vi "Variable@SDiff__Parameter.vi"(1 "ParamterIn":string) -> (0 "ParamterOut":string)   [LabVIEW 2020]
panel:
  out "f":i32
  in  "Var2":string(combo)
  in  "Section":string(combo)
  in  "Var1":string(combo)
  in  "ParameterName":string(combo)
  in  "Confirm":bool
  # "Variable@SUnion $Variable,$Var1,$Var2(,$Section)"
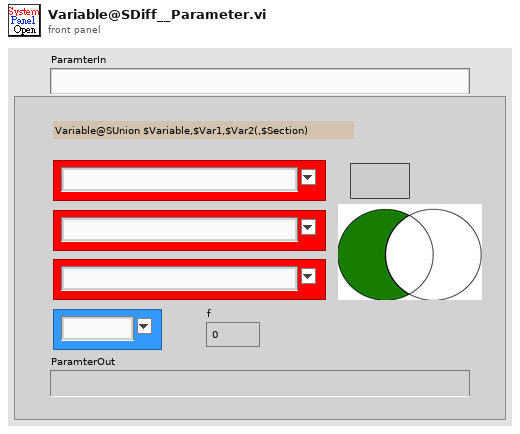
[diagram p1: front panel]
types:
  T1 = enum16{"Get", "Init", "Set", "Delete", "GetElement", "Inc", "Dec", "ReName"}
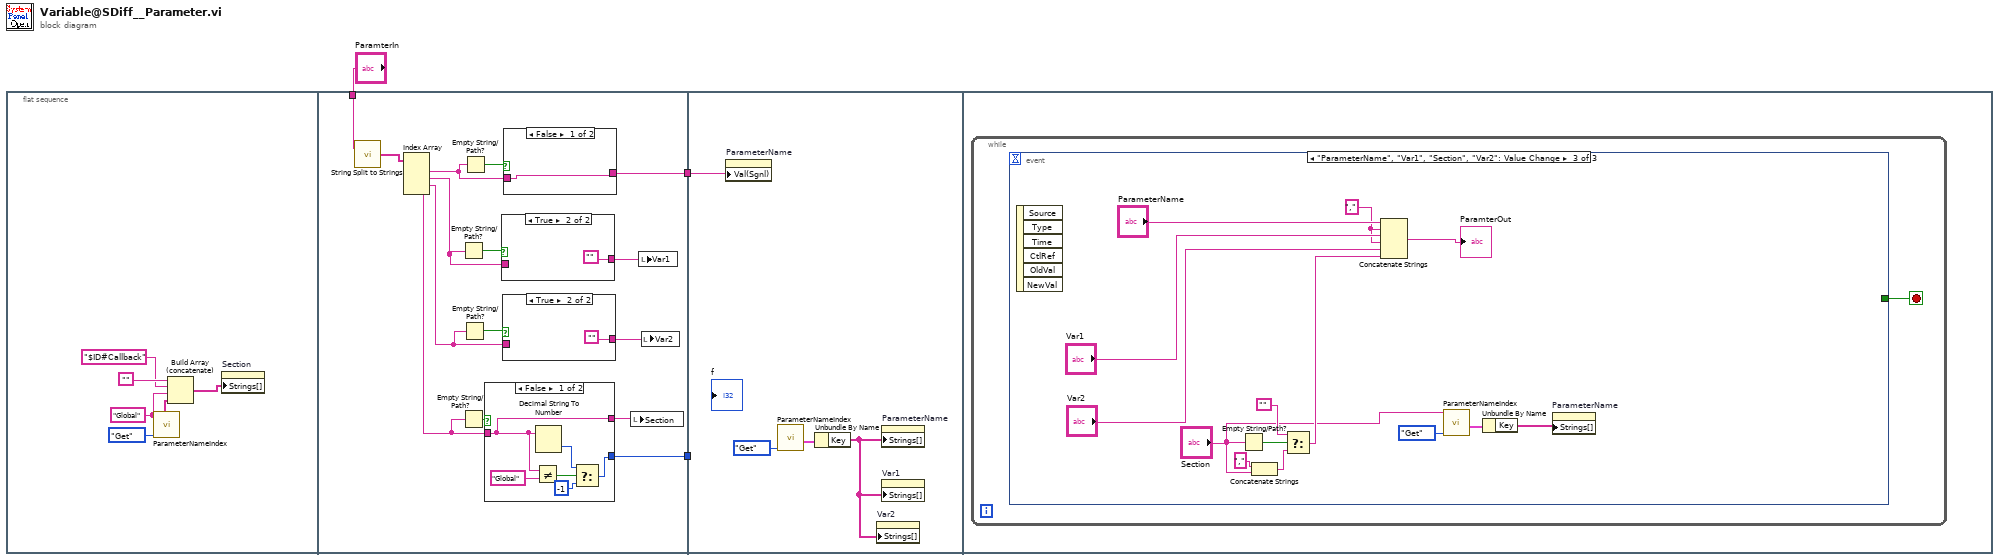
[diagram p0: block diagram]
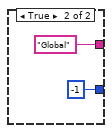
[diagram p3: hidden frame]
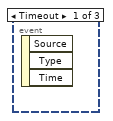
[diagram p6: hidden frame]
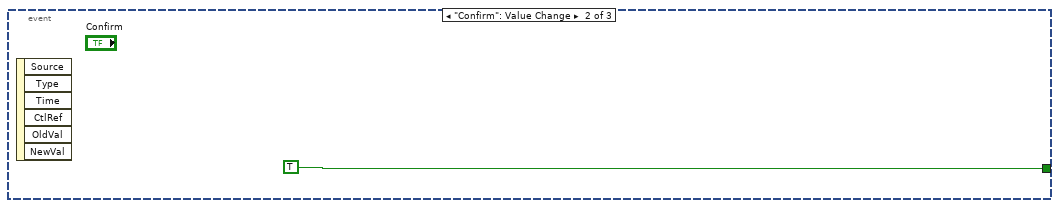
[diagram p7: hidden frame]
diagram:
  n1 = flat-sequence {
    tunnel: "ParamterIn" -> [w20]
    tunnel: [w22] -> w2
    tunnel: [w10] -> w1
    tunnel: w2 -> [w42]
    tunnel: w1 -> [_]
    frame #0 {
      w6 = "Global" ("VariableSection")
      n2 = call "ParameterNameIndex.vi"("OP"=T1."Get", "VariableSection"=w6) -> ("SectionList"=w7:string[])  [unwired: 3 in, 6 out]
      n3 = Build Array (concatenate)("", "$ID#Callback" ("VariableSection"), w6, w7) -> (w5:string[])
      n4 = property on="Section" class="CmbBox"("Strings[]"=w5) -> ()  [unwired: 2 in, 2 out]
    }
    frame #1 {
      n5 = call "String Split to Strings.vi"("String"=w20) -> ("Array"=w19:string[])  [unwired: 1 in]
      n6 = Index Array(array=w19) -> (element #1=w18:string, element #2=w17:string, element #3=w12:string, element #4=w15:string)  [unwired: 4 in]
      n7 = Empty String/Path?(string/path=w17) -> (empty?=w23:bool)
      n8 = Empty String/Path?(string/path=w15) -> (empty?=w16:bool)
      n9 = Empty String/Path?(string/path=w12) -> (empty?=w14:bool)
      n10 = Empty String/Path?(string/path=w18) -> (empty?=w24:bool)
      n11 = case shown="False" w16 {
        tunnel: w15 -> [w32 _]
        tunnel: [w32 "Global"] -> w11
        tunnel: [w27 -1] -> w10
        frame False {
          n12 = Not Equal?(x=w32, y="Global") -> (x != y?=w30:bool)
          n13 = Decimal String To Number(string=w32) -> (number=w29:i32)  [unwired: 2 in, 1 out]
          n14 = Select(t=w29, s=w30, f=-1) -> (s? t:f=w27:i32)
        }
        frame True {
        }
      }
      n15 = case shown="True" w23 {
        tunnel: w17 -> [w35 _]
        tunnel: [w35 ""] -> w21
        frame False {
        }
        frame True {
        }
      }
      n16 = case shown="True" w14 {
        tunnel: w12 -> [w25 _]
        tunnel: [w25 ""] -> w13
        frame False {
        }
        frame True {
        }
      }
      n17 = case shown="False" w24 {
        tunnel: w18 -> [w37 w38]
        tunnel: [w37 w38] -> w22
        frame False {
        }
        frame True {
        }
      }
      n18 = local write "Section"(w11) -> ()
      n19 = local write "Var1"(w21) -> ()
      n20 = local write "Var2"(w13) -> ()
    }
    frame #2 {
      n21 = property on="ParameterName" class="CmbBox"("Val(Sgnl)"=w42) -> ()  [unwired: 2 in, 2 out]
      n22 = call "ParameterNameIndex.vi"("OP"=T1."Get") -> ("GlobalKeyValue"=w40:cluster{"Key":string[], "Value":string[]})  [unwired: 4 in, 6 out]
      n23 = Unbundle By Name(w40) -> ("Key"=w41:string[])
      n24 = property on="Var2" class="CmbBox"("Strings[]"=w41) -> ()  [unwired: 2 in, 2 out]
      n25 = property on="ParameterName" class="CmbBox"("Strings[]"=w41) -> ()  [unwired: 2 in, 2 out]
      n26 = property on="Var1" class="CmbBox"("Strings[]"=w41) -> ()  [unwired: 2 in, 2 out]
    }
    frame #3 {
      n27 = while {
        stop <- w43 stop-if-true
        n28 = event shown="[2] \"ParameterName\", \"Var1\", \"Section\", \"Var2\": Value Change" {
          selector: _ -> [_ _ _]
          dyn-events: _ -> [_ _ _]
          timeout: _ -> [_ _ _]
          tunnel: [_ TRUE _] -> w43
          event Timeout {
            n29 = event-data() -> ()  [unwired: 1 in, 3 out]
          }
          event "Confirm": Value Change {
            n30 = event-data() -> ()  [unwired: 1 in, 6 out]
          }
          event "ParameterName", "Var1", "Section", "Var2": Value Change {
            w50 = "," ("string")
            n31 = event-data() -> ()  [unwired: 1 in, 6 out]
            n32 = Empty String/Path?(string/path="Section") -> (empty?=w54:bool)
            n33 = Concatenate Strings("," ("string"), "Section") -> (w55:string)
            n34 = Select(t="", s=w54, f=w55) -> (s? t:f=w48:string)
            n35 = Concatenate Strings("ParameterName", w50, "Var1", w50, "Var2", w48) -> (→"ParamterOut":string)
            n36 = call "ParameterNameIndex.vi"("OP"=T1."Get", "VariableSection"="Section") -> ("GlobalKeyValue"=w46:cluster{"Key":string[], "Value":string[]})  [unwired: 3 in, 6 out]
            n37 = Unbundle By Name(w46) -> ("Key"=w53:string[])
            n38 = property on="ParameterName" class="CmbBox"("Strings[]"=w53) -> ()  [unwired: 2 in, 2 out]
          }
        }
      }
    }
  }
